vi "trace v2.vi"(7 "pCtx":u32, 8 "error in (no error)":errorcluster, 9 "?":i32, 10 "uMask":u64, 11 "para0":dbl) -> (0 "error out":errorcluster, 2 "function return":i32, 3 "para0 out":dbl, 5 "pCtx out":u32)   [LabVIEW 2020, in "sqlite3.lvlib"]
uses:
  sqlite3.lvlib
  errstr.vi
  bin/sqlite3_64.dll
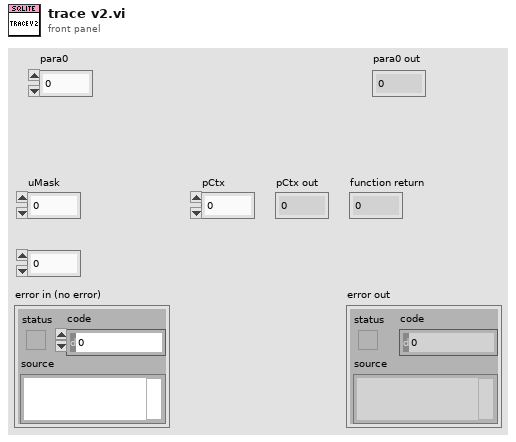
[diagram p1: front panel]
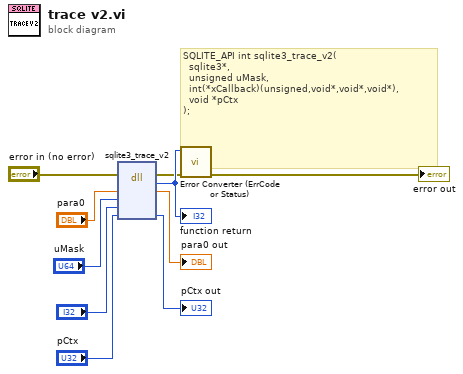
[diagram p0: block diagram]
diagram:
  # "SQLITE_API int sqlite3_trace_v2(\n  sqlite3*,\n  unsigned uMask,\n  int(*xCallback)(unsigned,void*,void*,void*),\n  void *pCtx\n);"
  n1 = dll-call lib="D:/Project/Labview-Projects/database-configuration/externals/sqlite3/Source/bin/sqlite3_*.*" fn="sqlite3_trace_v2"(error in="error in (no error)", "para0"="para0", "uMask"="uMask", "?", "pCtx"="pCtx") -> (error out=w2:errorcluster, w10:i32, "para0"=→"para0 out":dbl, "pCtx"=→"pCtx out":u32)  [unwired: 4 in, 1 out]
  "function return" <- w10
  n2 = call "Error Converter (ErrCode or Status).vi"("error in (no error)"=w2, "error code"=w10) -> ("error out"=→"error out":errorcluster)  [unwired: 9 in]
